vi "send load report.vi"(8 "error in":errorcluster, 9 "load error":errorcluster, 10 "engine loaded":string, 11 "message queue in":T1) -> (0 "error out":errorcluster, 3 "message queue out":T1)   [LabVIEW 2013, in "DCAF message service.lvlib"]
uses:
  DCAF message service.lvlib
  <vilib>/NI/AMC/Message Queue.ctl
  <vilib>/NI/AMC/Message.ctl
  <vilib>/NI/Tools/Keyed Array/KeyedArray.ctl
  common reponses to network process.ctl
  <vilib>/NI/AMC/Create Single Message.vi
  <vilib>/NI/AMC/Update Message Routing Info.vi
  <vilib>/NI/AMC/Send Message.vi
  <vilib>/NI/AMC/AMC.lvlib
  <vilib>/NI/Tools/Keyed Array/Tools_KeyedArray.lvlib
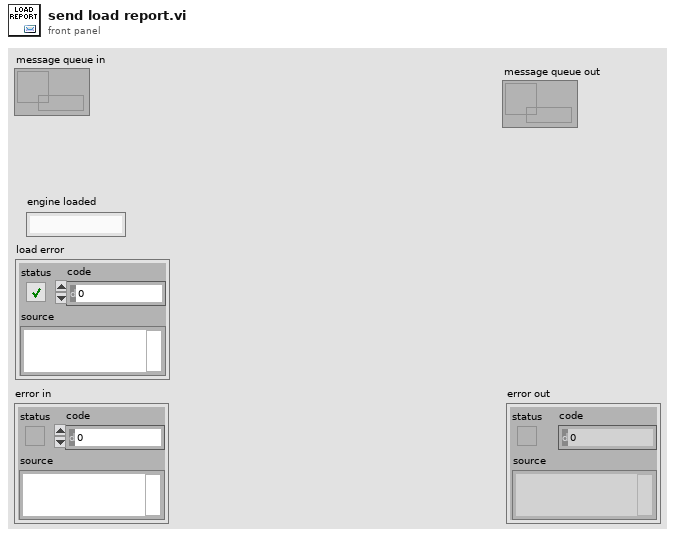
[diagram p1: front panel]
types:
  T1 = typedef "AMC.lvlib/Message Queue.ctl" = refnum<queue>
  T2 = cluster{"engine loaded":string, "load error":errorcluster}
  T3 = typedef "DCAF message service.lvlib/common reponses to network process.ctl" = enum16{"System Error", "Load Report", "Action Response", "Engine Status"}
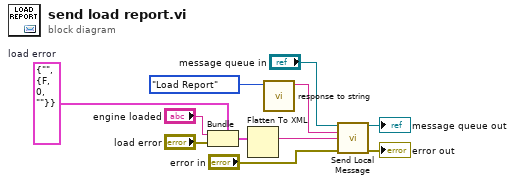
[diagram p0: block diagram]
diagram:
  w4 = T2 {"engine loaded"="", "load error"={"status"=FALSE, "code"=0, "source"=""}}  # load error
  n1 = Bundle(cluster=w4, "engine loaded"="engine loaded", "load error"="load error") -> (w3:T2)
  n2 = Flatten To XML(anything=w3) -> (xml string=w1:string)
  n3 = call "response to string.vi"("responses"=common_reponses_to_network_process."Load Report") -> ("command string"=w6:string)  [unwired: 10 in]
  n4 = call <vilib>:"Send Local Message.vi"("message queue in"="message queue in", "message name"=w6, "message value"=w1, "error in"="error in") -> ("message queue out"=→"message queue out":T1, "error out"=→"error out":errorcluster)  [unwired: 9 in, 1 out]
